vi "1D experiment kinect.vi"() -> ()   [LabVIEW 2011]
uses:
  <vilib>/Platform/TimedLoop/XDataNode/timing_clust.ctl
  <vilib>/Platform/TimedLoop/XDataNode/nitl_modes.ctl
  <vilib>/Platform/TimedLoop/XDataNode/wakeup.ctl
  <vilib>/Utility/inputDevices.llb/closeMouse.vi
  <vilib>/Utility/cursorutil.llb/Set Cursor (Cursor ID).vi
  <vilib>/Utility/inputDevices.llb/mouseAcquire.vi
  <vilib>/Utility/file.llb/Write To Spreadsheet File (DBL).vi
  <vilib>/Utility/file.llb/Write To Spreadsheet File (I64).vi
  <vilib>/Platform/TimedLoop/XDataNode/XDataNode.xnode
  <vilib>/Platform/TimedLoop/XDataNode/XDNodeRunTimeDep.lvlib
  User32.dll
  3D_Experiment/kinect-1-4/Kinect_API.lvlib
panel:
  in  "Far object filter 2":i32(slide)=26869 scale=0.0..4305.0
  out "click 2":bool
  in  "Replace with?":i32=60000
  out "stop":bool
  out "initial time":u32
  out "1D Experiment":cluster{"Y":dbl[], "Y":dbl[]}[](graph)
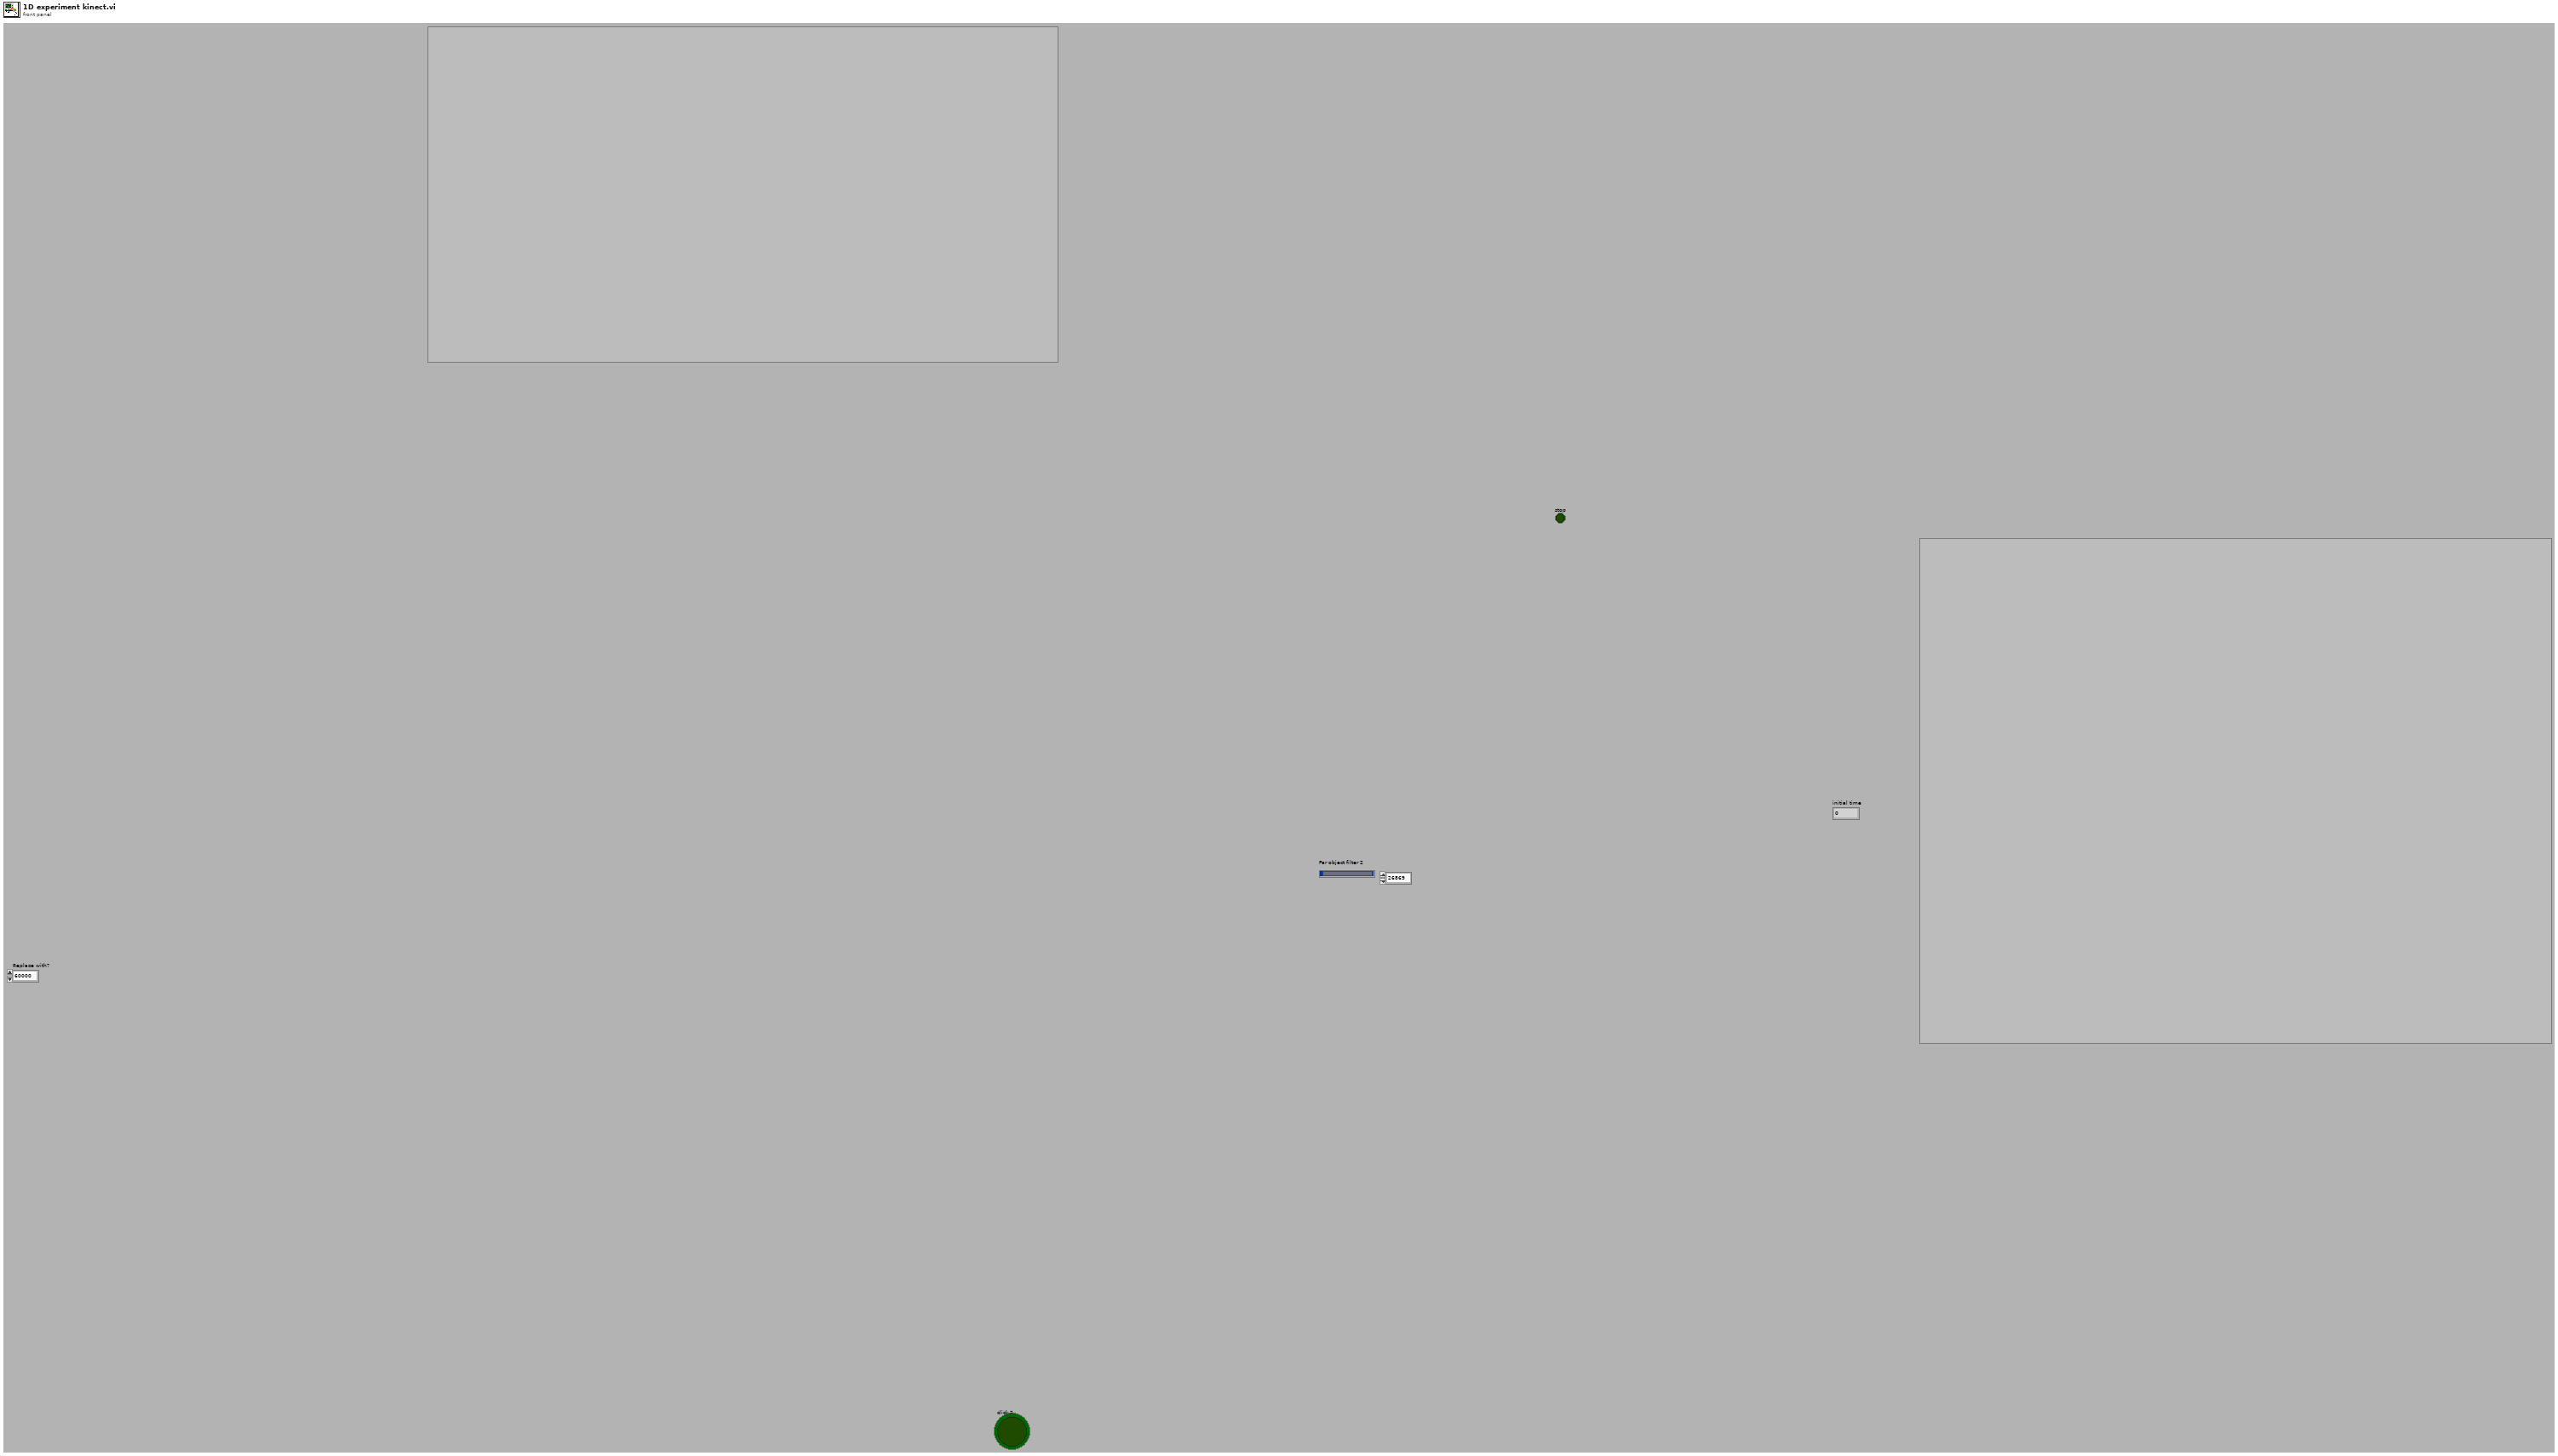
[diagram p1: front panel]
types:
  T1 = enum16{"open", "replace", "create", "open or create", "replace or create", "replace or create with confirmation"}
  T2 = typedef "XDNodeRunTimeDep.lvlib/timing_clust.ctl" = cluster{"Expected End [f-1]":u64, "Actual End [f-1]":u64, "Finished Late? [f-1]":bool, "Expected End [i-1]":u64, "Actual End [i-1]":u64, "Finished Late? [i-1]":bool, "Expected Start [i]":u64, "Actual Start [i]":u64, "Expected Start [f]":u64, "Actual Start [f]":u64, "Source Name":string, "Structure Name":string, "Period":i64, "Deadline":i64, "Offset":i64, "Start":i64, "Priority":i32, "Timeout":i32, "Mode":T3, "Wakeup Reason":T4, "Error":errorcluster, "Source Type":string, "Secondary Source Type":string, "Global End Time":u64, "Global Start Time":u64, "Frame Duration":u64, "Iteration Duration":u64, "Assigned CPU":i32, "I/O Scan Engine Mode":u32}
  T3 = typedef "XDNodeRunTimeDep.lvlib/nitl_modes.ctl" = enum32{"No Change", "Process missed periods, maintain original phase", "Discard missed periods, maintain original phase", "Process missed periods, ignore original phase", "Discard missed periods, ignore original phase"}
  T4 = typedef "XDNodeRunTimeDep.lvlib/wakeup.ctl" = enum32{"Normal", "Aborted", "Asynchronous wakeup", "Timing source error", "Timed loop error", "Timeout"}
  T5 = cluster{"Radius":dbl, "x0":dbl, "y0":dbl, "D":dbl, bool}
  T6 = typedef "LVAllMonitorsDisplayTypeDef.ctl" = cluster{"Bounds":cluster{"Left":i16, "Top":i16, "Right":i16, "Bottom":i16}, "Depth":i16}[]
  T7 = cluster{"Bounds":cluster{"Left":i16, "Top":i16, "Right":i16, "Bottom":i16}, "Depth":i16}
  T8 = cluster{"Left":i16, "Top":i16, "Right":i16, "Bottom":i16}
  T9 = cluster{"queue out":refnum<queue>, "queue out":refnum<queue>}
  T10 = cluster{"new reference":refnum<k24>, "DepthStream":refnum<k24>, "VideoStream":refnum<k24>, "Event Callback":refnum<k27>, "Event Callback":refnum<k27>}
  T11 = cluster{"Horizontal":i32, "Vertical":i32, "Scrolling":i32}
  T12 = cluster{"button 1":bool, "button 2":bool, "button 3":bool, "button 4":bool}
  T13 = typedef "LVPoint32TypeDef.ctl" = cluster{"Horizontal":i32, "Vertical":i32}
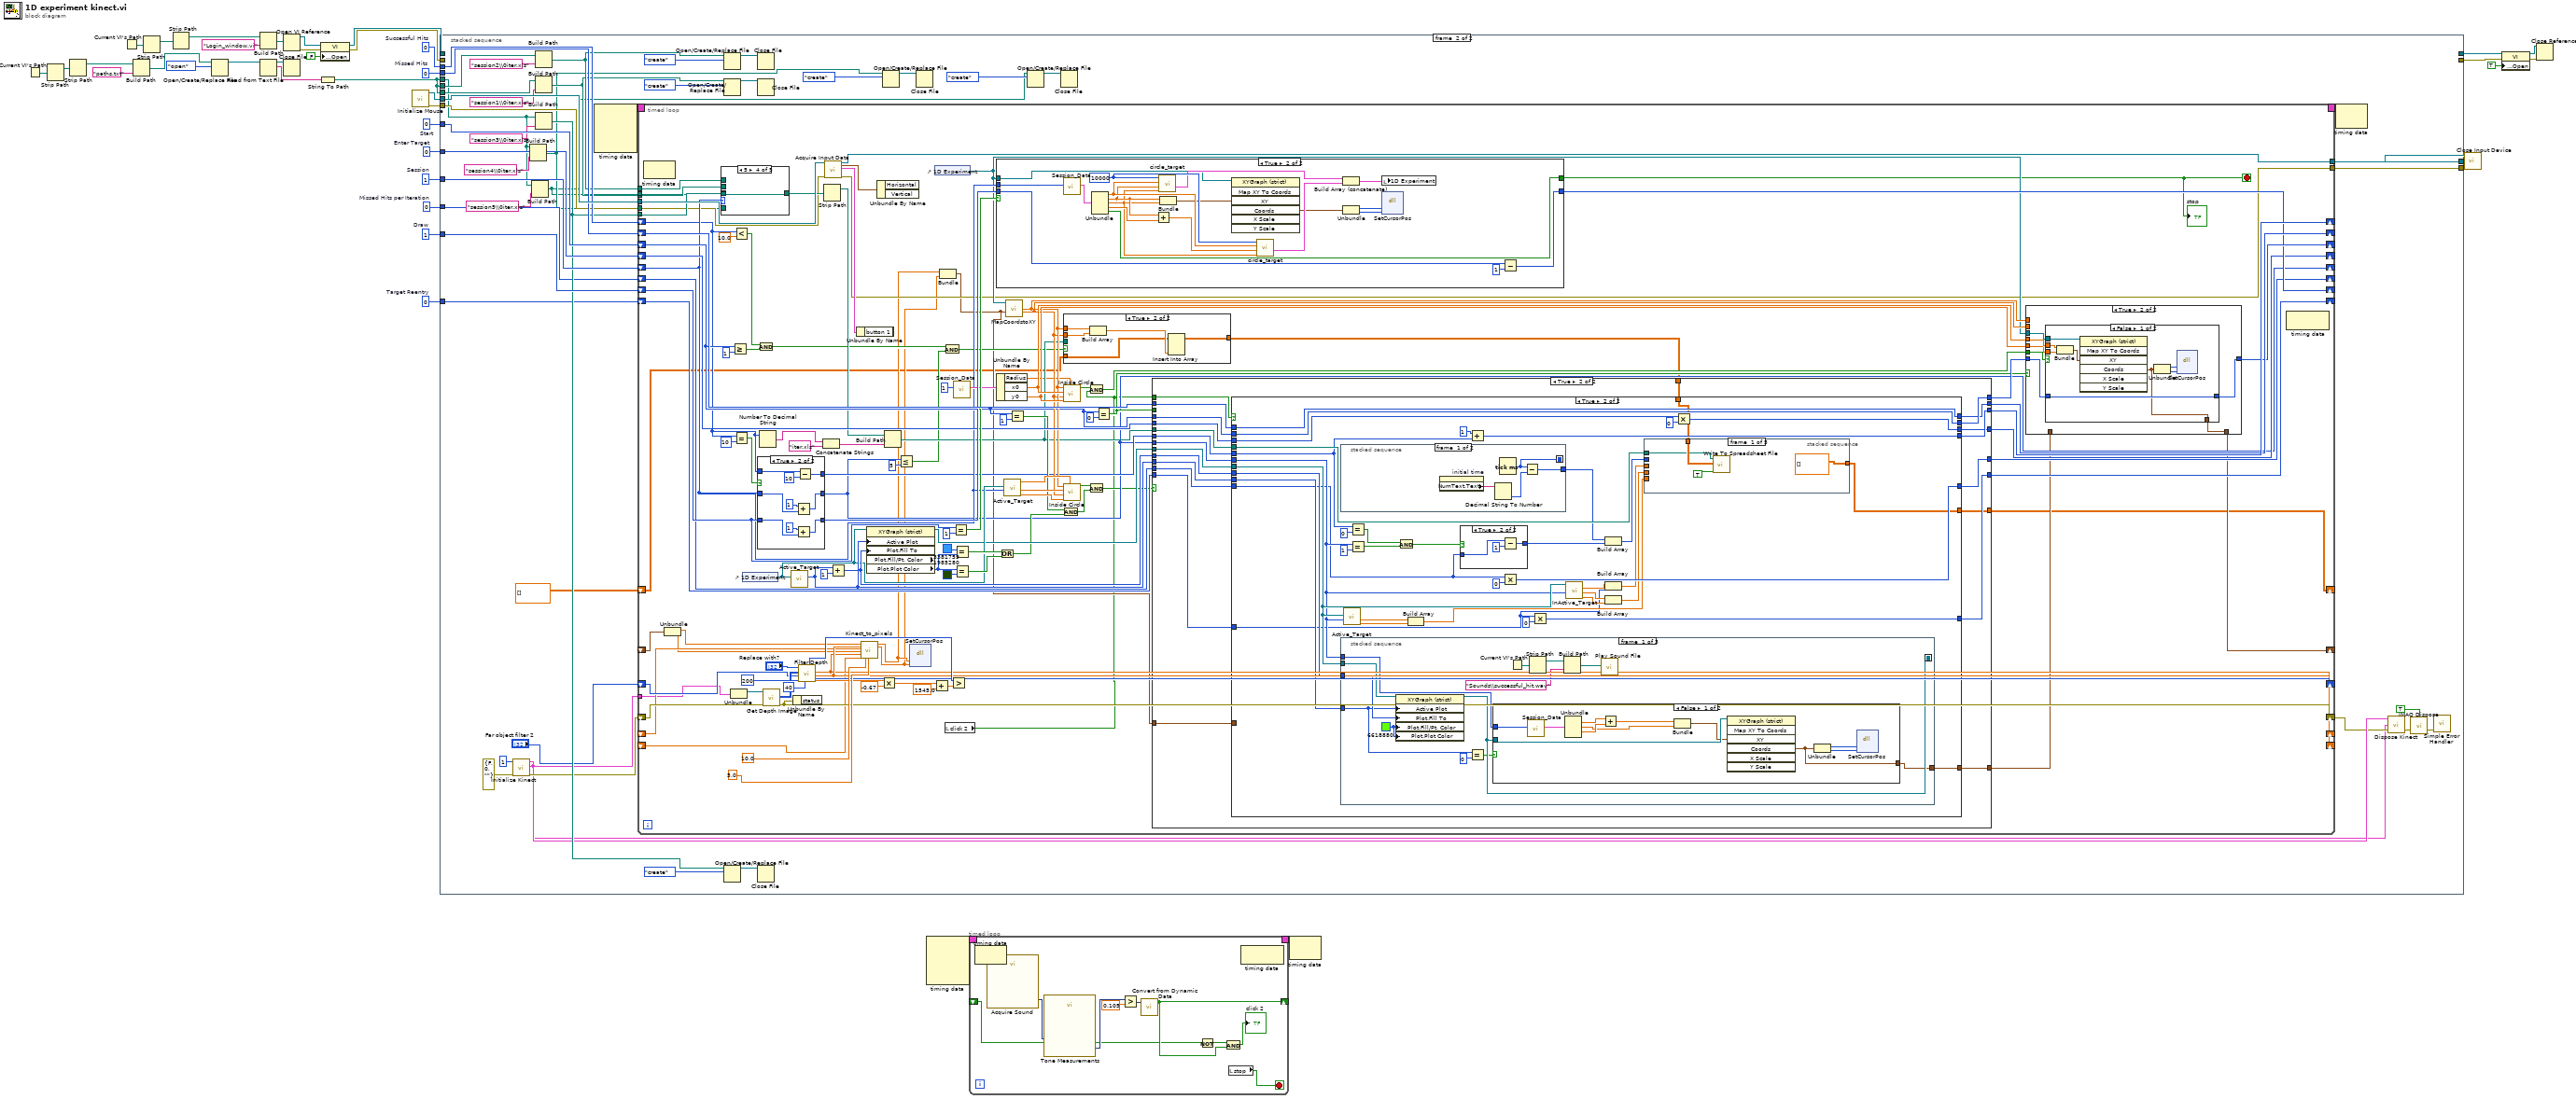
[diagram p0: block diagram]
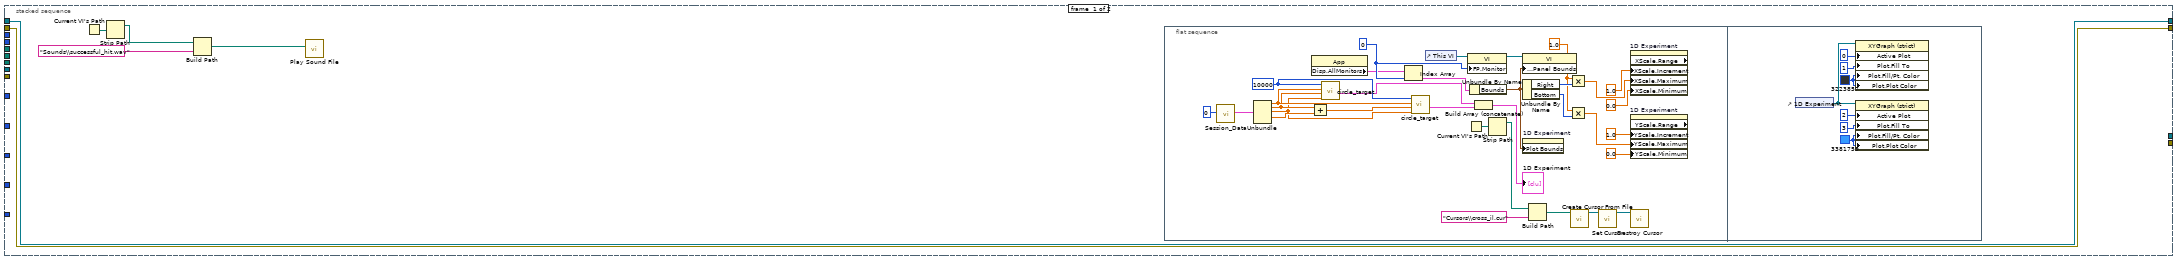
[diagram p2: hidden frame]
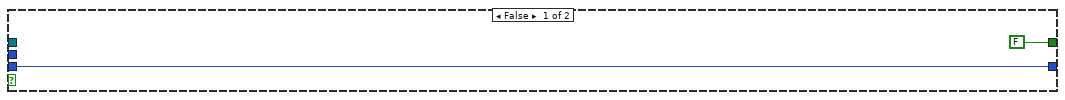
[diagram p8: hidden frame]
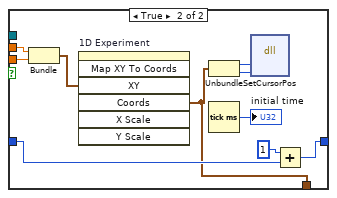
[diagram p10: hidden frame]
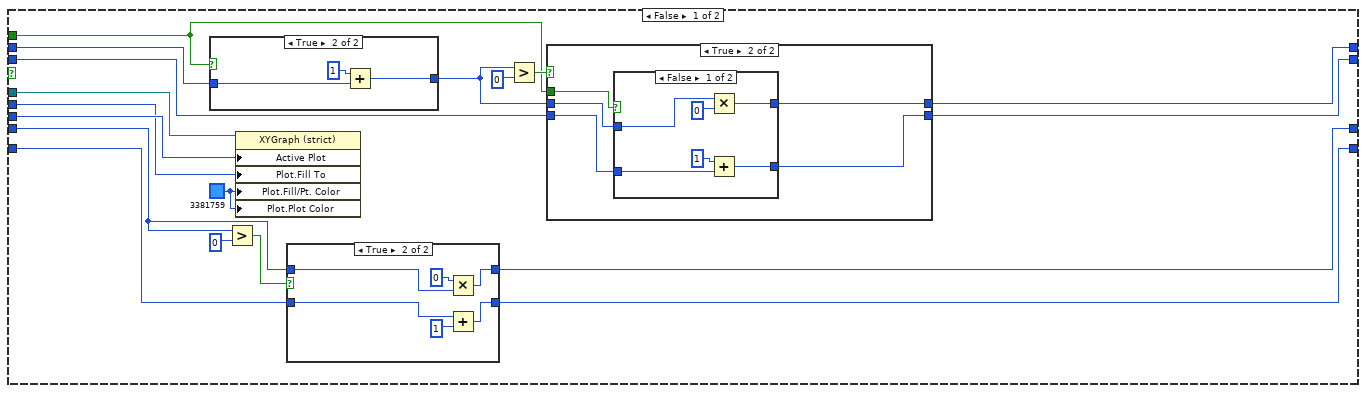
[diagram p13: hidden frame]
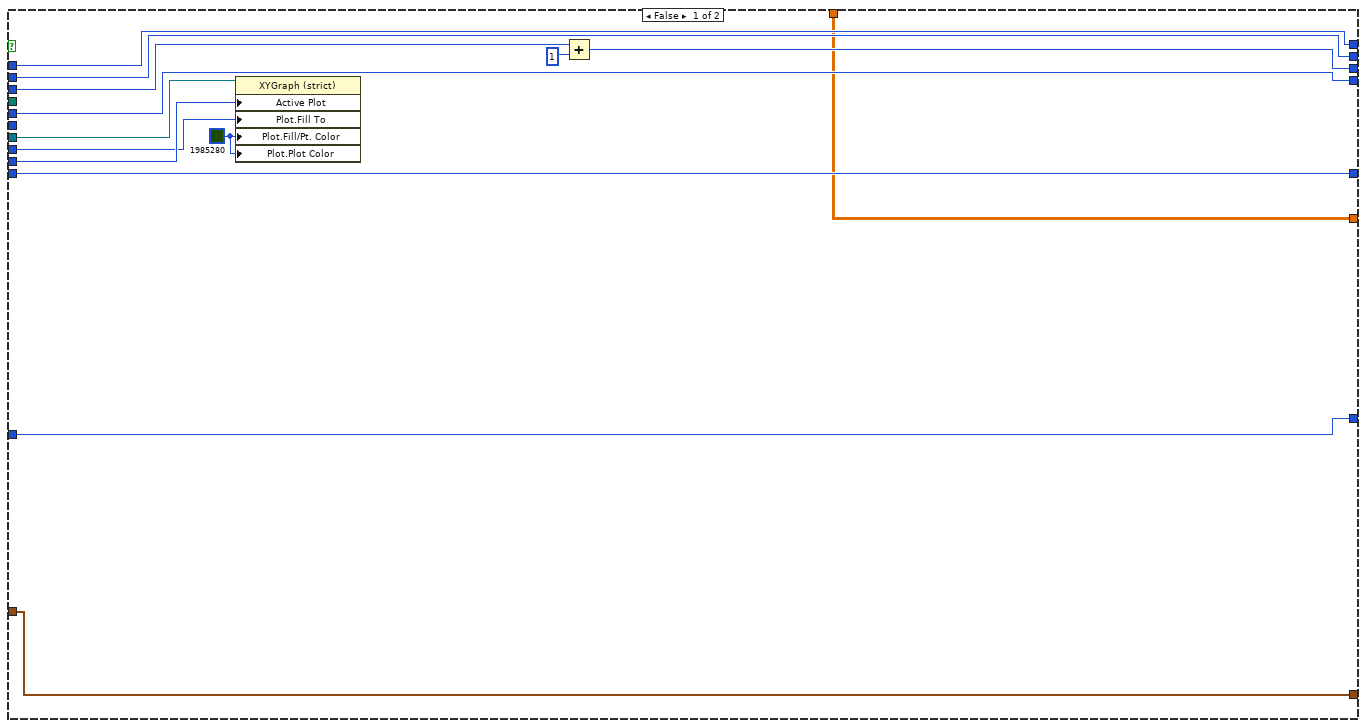
[diagram p18: hidden frame]
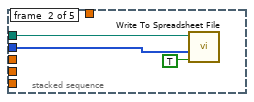
[diagram p20: hidden frame]
diagram:
  w5 = 0  # Target Reentry
  w6 = 0  # Missed Hits per Iteration
  w32 = 0  # Enter Target
  w33 = 1  # Draw
  w34 = 0  # Start
  w35 = 1  # Session
  w36 = 0  # Missed Hits
  w37 = 0  # Successful Hits
  n1 = Current VI's Path() -> (path=w14:path)
  n2 = Strip Path(path=w14) -> (stripped path=w9:path)  [unwired: 1 out]
  n3 = Strip Path(path=w9) -> (stripped path=w10:path)  [unwired: 1 out]
  n4 = Current VI's Path() -> (path=w17:path)
  n5 = Build Path(base path=w10, name or relative path="paths.txt") -> (appended path=w12:path)
  n6 = Strip Path(path=w17) -> (stripped path=w7:path)  [unwired: 1 out]
  n7 = Strip Path(path=w7) -> (stripped path=w8:path)  [unwired: 1 out]
  n8 = Open/Create/Replace File(file path (use dialog)=w12, operation (0:open)=T1."open") -> (refnum out=w30:refnum<file>)  [unwired: 4 in, 2 out]
  n9 = Build Path(base path=w8, name or relative path="Login_window.vi") -> (appended path=w15:path)
  n10 = Read from Text File(file (use dialog)=w30) -> (refnum out=w31:refnum<file>, text=w29:string)  [unwired: 3 in, 2 out]
  n11 = Open VI Reference(vi path=w15) -> (vi reference=w27:refnum<vi>, error out=w26:errorcluster)  [unwired: 5 in]
  n12 = Close File(refnum=w31) -> ()  [unwired: 1 in, 2 out]
  n13 = String To Path(string=w29) -> (path=w28:path)
  n14 = property class="VI"(reference=w27, error in=w26, "Front Panel Window:Open"=FALSE) -> (reference out=w24:refnum<vi>, error out=w23:errorcluster)
  n15 = call <vilib>:"Initialize Mouse.vi"() -> ("error out"=w4:errorcluster, "device ID"=w39:refnum<k1>)  [unwired: 1 in, 9 out]
  n16 = stacked-sequence {
    tunnel: w39 -> [_ w132]
    tunnel: [_ w131] -> w38
    tunnel: w37 -> [_ w130]
    tunnel: w36 -> [_ w129]
    tunnel: w35 -> [_ w125]
    tunnel: w34 -> [_ w128]
    tunnel: w33 -> [_ w127]
    tunnel: w32 -> [_ w126]
    tunnel: w28 -> [_ w115]
    tunnel: w28 -> [_ w122]
    tunnel: w28 -> [_ w102]
    tunnel: w24 -> [w41 _]
    tunnel: w23 -> [w40 _]
    tunnel: [w41 _] -> w19
    tunnel: [w40 _] -> w18
    tunnel: w6 -> [_ w108]
    tunnel: w5 -> [_ w107]
    tunnel: w4 -> [_ w106]
    tunnel: [_ w105] -> w3
    frame #0 {
      n17 = Current VI's Path() -> (path=w43:path)
      n18 = Strip Path(path=w43) -> (stripped path=w42:path)  [unwired: 1 out]
      n19 = Build Path(base path=w42, name or relative path="Sounds\\successful_hit.wav") -> (appended path=w44:path)
      n20 = call <vilib>:"Play Sound File.vi"("path"=w44) -> ()  [unwired: 9 in, 2 out]
      n21 = flat-sequence {
        frame #0 {
          w63 = 1.0 ("y")
          w68 = u16 0 ("Front Panel Window:Monitor")
          w77 = 10000
          n22 = call "Session_Data.vi"("Session"=0) -> ("output cluster"=w55:T5)  [unwired: 10 in]
          n23 = Unbundle(w55) -> ("Radius"=w75:dbl, "x0"=w53:dbl, "y0"=w52:dbl, "D"=w54:dbl)  [unwired: 1 out]
          n24 = Add(x=w53, y=w54) -> (x+y=w76:dbl)
          n25 = property class="App"() -> ("Disp.AllMonitors"=w67:T6)  [unwired: 2 in, 2 out]
          n26 = call "circle_target.vi"("y0"=w52, "x0"=w53, "Radius"=w75, "Pixels"=w77) -> ("Target plots"=w73:cluster{dbl[], dbl[]}[])  [unwired: 7 in]
          n27 = Index Array(array=w67, index=w68) -> (element=w69:T7)
          n28 = call "circle_target.vi"("y0"=w52, "x0"=w76, "Radius"=w75, "Pixels"=w77) -> ("Target plots"=w74:cluster{dbl[], dbl[]}[])  [unwired: 7 in]
          n29 = control-ref of="This VI"() -> (w70:refnum<vi>)
          n30 = Current VI's Path() -> (path=w51:path)
          n31 = property class="VI"(reference=w70, "FP.Monitor"=w68) -> (reference out=w66:refnum<vi>)  [unwired: 1 in, 1 out]
          n32 = Unbundle By Name(w69) -> ("Bounds"=w65:T8)
          n33 = Build Array (concatenate)(w73, w74) -> (→"1D Experiment":cluster{dbl[], dbl[]}[])
          n34 = Strip Path(path=w51) -> (stripped path=w50:path)  [unwired: 1 out]
          n35 = property class="VI"(reference=w66, "Front Panel Window:Panel Bounds"=w65) -> ()  [unwired: 1 in, 2 out]
          n36 = Unbundle By Name(w65) -> ("Right"=w64:i16, "Bottom"=w62:i16)
          n37 = property on="1D Experiment" class="XYGraph (strict)"("Plot Bounds"=w65) -> ()  [unwired: 2 in, 2 out]
          n38 = Build Path(base path=w50, name or relative path="Cursors\\cross_il.cur") -> (appended path=w48:path)
          n39 = Multiply(x=w63, y=w64) -> (x*y=w60:dbl)
          n40 = Multiply(x=w63, y=w62) -> (x*y=w57:dbl)
          n41 = call <vilib>:"Create Cursor From File.vi"("cursor file"=w48) -> ("cursor ID"=w47:refnum<k1>)  [unwired: 9 in, 1 out]
          n42 = call-poly <vilib>:"Set Cursor.vi"("cursor ID"=w47) -> ("previous cursor ID"=w46:refnum<k1>)  [unwired: 9 in, 1 out]
          n43 = property on="1D Experiment" class="XYGraph (strict)" props=["XScale", "Range", "XScale", "Increment", "XScale", "Maximum", "XScale", "Minimum"]("XScale.Increment"=1.0 ("X Scale.Range:Increment"), "XScale.Maximum"=w60, "XScale.Minimum"=0.0 ("X Scale.Range:Minimum")) -> ()  [unwired: 2 in, 3 out]
          n44 = property on="1D Experiment" class="XYGraph (strict)" props=["YScale", "Range", "YScale", "Increment", "YScale", "Maximum", "YScale", "Minimum"]("YScale.Increment"=1.0 ("Y Scale.Range:Increment"), "YScale.Maximum"=w57, "YScale.Minimum"=0.0 ("Y Scale.Range:Minimum")) -> ()  [unwired: 2 in, 3 out]
          n45 = call <vilib>:"Destroy Cursor.vi"("cursor ID"=w46) -> ()  [unwired: 9 in, 1 out]
        }
        frame #1 {
          w83 = u32 3381759
          w80 = u32 3223857
          n46 = control-ref of="1D Experiment"() -> (w84:refnum<vi>)
          n47 = property on="Property Node" class="XYGraph (strict)"(reference=w84, "Active Plot"=u32 0, "Plot.Fill To"=i16 1, "Plot.Fill/Pt. Color"=w80, "Plot.Plot Color"=w80) -> ()  [unwired: 1 in, 2 out]
          n48 = property on="Property Node" class="XYGraph (strict)"(reference=w84, "Active Plot"=u32 2, "Plot.Fill To"=i16 3, "Plot.Fill/Pt. Color"=w83, "Plot.Plot Color"=w83) -> ()  [unwired: 1 in, 2 out]
        }
      }
    }
    frame #1 {
      n49 = call "Initialize Kinect.vi"("error in (no error)"=errorcluster {"status"=FALSE, "code"=0, "source"=""}, "Buffer Size"=1) -> ("error out"=w93:errorcluster, "Queues Out"=w86:T9, "References"=w88:T10)  [unwired: 7 in]
      n50 = Build Path(base path=w102, name or relative path="session4\\0iter.xls") -> (appended path=w97:path)
      n51 = Build Path(base path=w102, name or relative path="session5\\0iter.xls") -> (appended path=w96:path)
      n52 = Build Path(base path=w122, name or relative path="session2\\0iter.xls") -> (appended path=w119:path)
      n53 = Build Path(base path=w115, name or relative path="session1\\0iter.xls") -> (appended path=w111:path)
      n54 = Build Path(base path=w102, name or relative path="session3\\0iter.xls") -> (appended path=w116:path)
      n55 = node-c288() -> (w110:T2)  [unwired: 4 in]
      n56 = timed-loop {
        tunnel: w132 -> [w236]
        tunnel: [w235] -> w131
        shift-right: [w233] -> _
        shift-left: w130 -> [w185]
        shift-right: [w231] -> _
        shift-left: w129 -> [w232]
        shift-right: [w176] -> _
        shift-left: w125 -> [w198]
        shift-right: [w223] -> _
        shift-left: w128 -> [w201]
        shift-right: [w217] -> _
        shift-left: w127 -> [w218]
        shift-right: [w213] -> _
        shift-left: w126 -> [w214]
        tunnel: w111 -> [w199]
        tunnel: w119 -> [w197]
        tunnel: w116 -> [w196]
        timing: w110 -> [_]
        timing-out: [_] -> w109
        shift-right: [w181] -> _
        shift-left: w108 -> [w183]
        shift-right: [w179] -> _
        shift-left: w107 -> [w180]
        tunnel: w106 -> [w171]
        tunnel: [w170] -> w105
        tunnel: w97 -> [w169]
        tunnel: w96 -> [w168]
        shift-right: [w153] -> _
        shift-left: "Far object filter 2" -> [w152]
        shift-right: [w151] -> w87
        shift-left: w93 -> [w150]
        shift-right: [w149] -> _
        shift-left: _ -> [w148]
        shift-right: [w147] -> _
        shift-left: _ -> [w146]
        tunnel: w86 -> [w145]
        shift-right: [w142] -> _
        shift-left: _ -> [w141]
        shift-right: [w133] -> _
        shift-left: dbl[][] [] -> [w135]
        stop <- w167 stop-if-true
        n57 = node-c288() -> ()  [unwired: 1 in, 1 out]
        n58 = Unbundle(w141) -> ("X_pixels"=w140:dbl, "Y_pixels"=w139:dbl)
        n59 = case shown="5" w198 {
          tunnel: w199 -> [_ _ _ _ w253]
          tunnel: [w249 w250 w251 w252 w253] -> w194
          tunnel: w197 -> [w249 _ _ _ _]
          tunnel: w196 -> [_ w250 _ _ _]
          tunnel: w169 -> [_ _ w251 _ _]
          tunnel: w168 -> [_ _ _ w252 _]
          frame 2 {
          }
          frame 3 {
          }
          frame 4 {
          }
          frame 5 {
          }
          frame 1, Default {
          }
        }
        n60 = Unbundle(w145) -> ("queue out"=w154:refnum<queue>)  [unwired: 1 out]
        n61 = Greater Or Equal?(x=w201, y=1) -> (x >= y?=w188:bool)
        n62 = Less?(x=w185, y=10.0) -> (x < y?=w187:bool)
        n63 = Equal?(x=w185, y=10) -> (x = y?=w229:bool)
        n64 = control-ref of="1D Experiment"() -> (w227:refnum<vi>)
        n65 = case shown="True" w229 {
          tunnel: w185 -> [w311 w320]
          tunnel: [w311 w318] -> w195
          tunnel: w198 -> [w310 w312]
          tunnel: [w310 w313] -> w176
          tunnel: w218 -> [w309 w316]
          tunnel: [w309 w314] -> w216
          frame False {
          }
          frame True {
            n66 = Add(x=1, y=w312) -> (x+y=w313:i32)
            n67 = Add(x=1, y=w316) -> (x+y=w314:i32)
            n68 = Subtract(x=w320, y=10) -> (x-y=w318:i32)
          }
        }
        n69 = And(x=w187, y=w188) -> (x .and. y?=w177:bool)
        n70 = Number To Decimal String(number=w185) -> (decimal integer string=w193:string)  [unwired: 1 in]
        n71 = call "Get Depth Image.vi"("error in (no error)"=w150, "queue in"=w154) -> ("error out"=w151:errorcluster, "Depth Image Pixels (U16)"=w156:u16[][])  [unwired: 6 in, 2 out]
        n72 = call "Active_Target.vi"("XYGraph Refnum"=w227) -> ("Active Plot"=w241:u32)  [unwired: 7 in, 3 out]
        n73 = Unbundle By Name(w151) -> ()  [unwired: 1 out]
        n74 = call "Filter Depth.vi"("Wall-Threshold"=40, "Y-Threshold"=200, "Far object filter"=w152, "Depth Image Pixels (U16)"=w156, "Replace with?"="Replace with?") -> ("average Z"=w162:dbl, "average Y"=w149:dbl, "average X"=w147:dbl, "New far object filter"=w153:i32, "Area"=w163:i32)  [unwired: 1 in, 1 out]
        n75 = Concatenate Strings(w193, "iter.xls" ("name or relative path")) -> (w191:string)
        n76 = Strip Path(path=w194) -> (stripped path=w190:path)  [unwired: 1 out]
        n77 = call-poly <vilib>:"Acquire Input Data.vi"("device ID"=w236, "error in (no error)"=w171) -> ("device ID"=w235:refnum<k1>, "axis info"=w234:T11, "button info"=w237:T12, "error out"=w170:errorcluster)  [unwired: 1 in, 13 out]
        n78 = Add(x=w241, y=u32 1) -> (x+y=w240:u32)
        n79 = Unbundle By Name(w237) -> ()  [unwired: 1 out]
        n80 = call "Kinect_to_pixels.vi"("previous_X_pixels"=w140, "current_X_kinect"=w149, "previous_X_kinect"=w148, "previous_Y_pixels"=w139, "current_Y_kinect"=w147, "previous_Y_kinect"=w146, "X_Y_speed"=10.0, "min_diff"=5.0) -> ("X_pixels"=w138:dbl, "Y_pixels"=w137:dbl)  [unwired: 8 in, 2 out]
        n81 = property on="Property Node" class="XYGraph (strict)" props=["Active Plot", "Plot", "Fill To", "Plot", "Fill/Pt. Color", "Plot", "Plot Color"](reference=w227, "Active Plot"=w241, "Plot.Fill To"=w240) -> (reference out=w220:refnum<vi>, "Plot.Plot Color"=w222:u32)  [unwired: 1 in, 2 out]
        n82 = Unbundle By Name(w234) -> ()  [unwired: 2 out]
        n83 = Multiply(x=w162, y=-0.67 ("x")) -> (x*y=w158:dbl)
        n84 = Build Path(base path=w190, name or relative path=w191) -> (appended path=w189:path)
        n85 = Less Or Equal?(x=w176, y=5) -> (x <= y?=w173:bool)
        n86 = dll-call lib="User32.dll" fn="SetCursorPos"(w138, w137) -> ()  [unwired: 6 in, 2 out]
        n87 = Add(x=w158, y=1545.0 ("x")) -> (x+y=w159:dbl)
        n88 = control-ref of="1D Experiment"() -> (w184:refnum<vi>)
        n89 = Bundle("X_pixels"=w138, "Y_pixels"=w137) -> (w143:cluster{"X_pixels":dbl, "Y_pixels":dbl})  [unwired: 1 in]
        n90 = And(x=w177, y=w173) -> (x .and. y?=w174:bool)
        n91 = local read "click 2"() -> (w136:bool)
        n92 = Greater?(x=w163, y=w159) -> ()  [unwired: 1 out]
        n93 = Equal?(x=w218, y=1) -> (x = y?=w215:bool)
        n94 = call "Session_Data.vi"("Session"=1) -> ("output cluster"=w207:T5)  [unwired: 10 in]
        n95 = Equal?(x=u32 3381759, y=w222) -> (x = y?=w244:bool)
        n96 = Equal?(x=w222, y=u32 1985280) -> (x = y?=w243:bool)
        n97 = case shown="True" w215 {
          tunnel: w198 -> [_ w270]
          tunnel: [w260 w280] -> w217
          tunnel: w216 -> [w260 w279]
          tunnel: [FALSE ("Valid") w269] -> w167
          tunnel: w184 -> [_ w265]
          frame False {
          }
          frame True {
            w278 = 10000
            n98 = call "Session_Data.vi"("Session"=w270) -> ("output cluster"=w273:T5)  [unwired: 10 in]
            n99 = Unbundle(w273) -> ("Radius"=w276:dbl, "x0"=w264:dbl, "y0"=w263:dbl, "D"=w272:dbl, w269:bool)
            n100 = Add(x=w264, y=w272) -> (x+y=w277:dbl)
            n101 = call "circle_target.vi"("y0"=w263, "x0"=w264, "Radius"=w276, "Pixels"=w278) -> ("Target plots"=w274:cluster{dbl[], dbl[]}[])  [unwired: 7 in]
            n102 = Bundle("x0"=w264, "y0"=w263) -> (w262:cluster{"x0":dbl, "y0":dbl})  [unwired: 1 in]
            n103 = invoke on="Invoke Node" class="XYGraph (strict)" method="Map XY To Coords"(reference=w265, "XY"=w262) -> ("Coords"=w268:T13)  [unwired: 5 in, 6 out]
            n104 = call "circle_target.vi"("y0"=w263, "x0"=w277, "Radius"=w276, "Pixels"=w278) -> ("Target plots"=w275:cluster{dbl[], dbl[]}[])  [unwired: 7 in]
            n105 = Build Array (concatenate)(w274, w275) -> (w271:cluster{dbl[], dbl[]}[])
            n106 = Unbundle(w268) -> ("Horizontal"=w267:i32, "Vertical"=w266:i32)
            n107 = local write "1D Experiment"(w271) -> ()
            n108 = dll-call lib="User32.dll" fn="SetCursorPos"(w267, w266) -> ()  [unwired: 6 in, 2 out]
            n109 = Subtract(x=w279, y=1) -> (x-y=w280:i32)
          }
        }
        "stop" <- w167
        n110 = Unbundle By Name(w207) -> ("Radius"=w178:dbl, "x0"=w206:dbl, "y0"=w205:dbl)
        n111 = Or(x=w244, y=w243) -> (x .or. y?=w211:bool)
        n112 = call "Active_Target.vi"("Session"=w198, "XYGraph Refnum"=w227) -> ("y0"=w238:dbl, "x0"=w239:dbl, "Radius"=w228:dbl)  [unwired: 6 in, 1 out]
        n113 = call "MapCoordstoXY.vi"("Coordinates"=w143, "XYGraph Refnum"=w184) -> ("Y(graph)"=w202:dbl, "X (graph)"=w203:dbl)  [unwired: 7 in]
        n114 = Equal?(x=w201, y=1) -> (x = y?=w209:bool)
        n115 = And(x=w209, y=w211) -> (x .and. y?=w208:bool)
        n116 = case shown="True" w174 {
          tunnel: w203 -> [_ w259]
          tunnel: w202 -> [_ w258]
          tunnel: w189 -> [_ _]
          tunnel: w135 -> [w254 w256]
          tunnel: [w254 w255] -> w134
          frame False {
          }
          frame True {
            n117 = Build Array(w259, w258) -> (w257:dbl[])
            n118 = Insert Into Array(array=w256, new element=w257) -> (w255:dbl[][])  [unwired: 2 in]
          }
        }
        n119 = call "Inside Circle.vi"("Radius"=w178, "y0"=w205, "y"=w202, "x0"=w206, "x"=w203) -> ("Inside Circle"=w225:bool)  [unwired: 6 in]
        n120 = call "Inside Circle.vi"("Radius"=w228, "y0"=w238, "y"=w202, "x0"=w239, "x"=w203) -> ("Inside Circle"=w210:bool)  [unwired: 6 in]
        n121 = And(x=w225, y=w136) -> (x .and. y?=w224:bool)
        n122 = And(x=w210, y=w208) -> (x .and. y?=w172:bool)
        n123 = Equal?(x=w201, y=0) -> (x = y?=w182:bool)
        n124 = case shown="True" w172 {
          tunnel: w136 -> [w331 w408]
          tunnel: w241 -> [w335 w405]
          tunnel: w240 -> [w334 w404]
          tunnel: w195 -> [w337 w407]
          tunnel: [w337 w406] -> w233
          tunnel: w232 -> [w336 w396]
          tunnel: [w328 w394] -> w231
          tunnel: w201 -> [w333 w403]
          tunnel: [w333 w402] -> w221
          tunnel: w220 -> [w332 w401]
          tunnel: w214 -> [w326 w400]
          tunnel: [w325 w399] -> w213
          tunnel: w176 -> [_ w398]
          tunnel: w189 -> [_ w397]
          tunnel: w183 -> [w330 w395]
          tunnel: w182 -> [w329 _]
          tunnel: [w327 w393] -> w181
          tunnel: w180 -> [w324 w392]
          tunnel: [w323 w391] -> w179
          tunnel: [w322 w390] -> w144
          tunnel: w143 -> [w322 w389]
          tunnel: w134 -> [w321 w388]
          tunnel: [w321 w387] -> w133
          frame False {
            n125 = case shown="True" w329 {
              tunnel: w336 -> [w354 w385]
              tunnel: w335 -> [w353 _]
              tunnel: w334 -> [w352 _]
              tunnel: w332 -> [w351 _]
              tunnel: w331 -> [w348 _]
              tunnel: w330 -> [w346 w386]
              tunnel: [w345 w385] -> w328
              tunnel: [w344 w386] -> w327
              tunnel: w326 -> [w341 w384]
              tunnel: [w340 w384] -> w325
              tunnel: w324 -> [w339 w383]
              tunnel: [w338 w383] -> w323
              frame False {
                w355 = u32 3381759
                n126 = case shown="True" w348 {
                  tunnel: w354 -> [w379 w382]
                  tunnel: [w379 w380] -> w347
                  frame False {
                  }
                  frame True {
                    n127 = Add(x=1, y=w382) -> (x+y=w380:i32)
                  }
                }
                n128 = Greater?(x=w341, y=0) -> (0:w342:bool)
                n129 = property on="Property Node" class="XYGraph (strict)"(reference=w351, "Active Plot"=w353, "Plot.Fill To"=w352, "Plot.Fill/Pt. Color"=w355, "Plot.Plot Color"=w355) -> ()  [unwired: 1 in, 2 out]
                n130 = case shown="True" w342 {
                  tunnel: w341 -> [w357 w363]
                  tunnel: [w357 w361] -> w340
                  tunnel: w339 -> [w356 w360]
                  tunnel: [w356 w358] -> w338
                  frame False {
                  }
                  frame True {
                    n131 = Multiply(x=0, y=w363) -> (x*y=w361:i32)
                    n132 = Add(x=w360, y=1) -> (x+y=w358:i32)
                  }
                }
                n133 = Greater?(x=w347, y=0) -> (0:w349:bool)
                n134 = case shown="True" w349 {
                  tunnel: [w364 w370] -> w344
                  tunnel: [w365 w369] -> w345
                  tunnel: w348 -> [_ w368]
                  tunnel: w347 -> [w365 w367]
                  tunnel: w346 -> [w364 w366]
                  frame False {
                  }
                  frame True {
                    n135 = case shown="False" w368 {
                      tunnel: [w375 w378] -> w370
                      tunnel: [w373 w377] -> w369
                      tunnel: w367 -> [w372 w377]
                      tunnel: w366 -> [w371 w378]
                      frame False {
                        n136 = Multiply(x=w372, y=0) -> (x*y=w373:i32)
                        n137 = Add(x=1, y=w371) -> (x+y=w375:i32)
                      }
                      frame True {
                      }
                    }
                  }
                }
              }
              frame True {
              }
            }
          }
          frame True {
            n138 = case shown="True" w408 {
              tunnel: w407 -> [w421 w436]
              tunnel: [w421 w456] -> w406
              tunnel: w405 -> [w420 w459]
              tunnel: w404 -> [w419 w458]
              tunnel: w403 -> [w417 w457]
              tunnel: [w417 w457] -> w402
              tunnel: w401 -> [w418 w443]
              tunnel: w400 -> [w413 w448]
              tunnel: [w414 w446] -> w399
              tunnel: w398 -> [_ w434]
              tunnel: w397 -> [_ w454]
              tunnel: w396 -> [w416 w452]
              tunnel: [w416 w452] -> w394
              tunnel: w395 -> [w415 w429]
              tunnel: [w415 w450] -> w393
              tunnel: w392 -> [w411 w427]
              tunnel: [w411 w445] -> w391
              tunnel: [w410 w425] -> w390
              tunnel: w389 -> [w410 _]
              tunnel: w388 -> [w409 w424]
              tunnel: [w409 w423] -> w387
              frame False {
                w422 = u32 1985280
                n139 = property on="Property Node" class="XYGraph (strict)"(reference=w418, "Active Plot"=w420, "Plot.Fill To"=w419, "Plot.Fill/Pt. Color"=w422, "Plot.Plot Color"=w422) -> ()  [unwired: 1 in, 2 out]
                n140 = Add(x=w413, y=1) -> (x+y=w414:i32)
              }
              frame True {
                n141 = stacked-sequence {
                  seq-local: [w481 _] -> [_ w485]
                  tunnel: [w482 _] -> w453
                  frame #0 {
                    n142 = property on="initial time" class="DigNum (strict)"() -> ("NumText.Text"=w484:string)  [unwired: 2 in, 2 out]
                    n143 = Decimal String To Number(string=w484) -> (number=w483:i32)  [unwired: 2 in, 1 out]
                    n144 = Tick Count (ms)() -> (millisecond timer value=w481:u32)
                    n145 = Subtract(x=w481, y=w483) -> (x-y=w482:u32)
                  }
                  frame #1 {
                    n146 = Number To Decimal String(number=w485) -> (decimal integer string=w486:string)  [unwired: 1 in]
                    n147 = property on="initial time" class="DigNum (strict)"("NumText.Text"=w486) -> ()  [unwired: 2 in, 2 out]
                  }
                }
                n148 = stacked-sequence {
                  seq-local: [w496 _ _] -> [_ w520 w529]
                  tunnel: w459 -> [w495 w521 w531]
                  tunnel: w458 -> [w498 _ w530]
                  tunnel: w443 -> [w497 _ _]
                  tunnel: w434 -> [w492 _ _]
                  tunnel: [w487 _ _] -> w425
                  frame #0 {
                    w499 = u32 6618880
                    n149 = property on="Property Node" class="XYGraph (strict)"(reference=w497, "Active Plot"=w495, "Plot.Fill To"=w498, "Plot.Fill/Pt. Color"=w499, "Plot.Plot Color"=w499) -> (reference out=w496:refnum<vi>)  [unwired: 1 in, 1 out]
                    n150 = Equal?(x=w495, y=u32 0) -> (x = y?=w493:bool)
                    n151 = case shown="False" w493 {
                      tunnel: w496 -> [w507 w513]
                      tunnel: w492 -> [w505 w517]
                      tunnel: [w500 w511] -> w487
                      frame False {
                        n152 = call "Session_Data.vi"("Session"=w505) -> ("output cluster"=w508:T5)  [unwired: 10 in]
                        n153 = Unbundle(w508) -> ("x0"=w503:dbl, "y0"=w501:dbl, "D"=w502:dbl)  [unwired: 2 out]
                        n154 = Add(x=w503, y=w502) -> (x+y=w504:dbl)
                        n155 = Bundle(w504, "y0"=w501) -> (w506:cluster{dbl, "y0":dbl})  [unwired: 1 in]
                        n156 = invoke on="Invoke Node" class="XYGraph (strict)" method="Map XY To Coords"(reference=w507, "XY"=w506) -> ("Coords"=w500:T13)  [unwired: 5 in, 6 out]
                        n157 = Unbundle(w500) -> ("Horizontal"=w510:i32, "Vertical"=w509:i32)
                        n158 = dll-call lib="User32.dll" fn="SetCursorPos"(w510, w509) -> ()  [unwired: 6 in, 2 out]
                      }
                      frame True {
                        n159 = call "Session_Data.vi"("Session"=w517) -> ("output cluster"=w516:T5)  [unwired: 10 in]
                        n160 = Unbundle(w516) -> ("x0"=w515:dbl, "y0"=w512:dbl)  [unwired: 3 out]
                        n161 = Bundle("x0"=w515, "y0"=w512) -> (w514:cluster{"x0":dbl, "y0":dbl})  [unwired: 1 in]
                        n162 = invoke on="Invoke Node" class="XYGraph (strict)" method="Map XY To Coords"(reference=w513, "XY"=w514) -> ("Coords"=w511:T13)  [unwired: 5 in, 6 out]
                        n163 = Unbundle(w511) -> ("Horizontal"=w519:i32, "Vertical"=w518:i32)
                        n164 = dll-call lib="User32.dll" fn="SetCursorPos"(w519, w518) -> ()  [unwired: 6 in, 2 out]
                      }
                    }
                    n165 = Current VI's Path() -> (path=w489:path)
                    n166 = Strip Path(path=w489) -> (stripped path=w488:path)  [unwired: 1 out]
                    n167 = Build Path(base path=w488, name or relative path="Sounds\\successful_hit.wav") -> (appended path=w490:path)
                    n168 = call <vilib>:"Play Sound File.vi"("path"=w490) -> ()  [unwired: 9 in, 2 out]
                  }
                  frame #1 {
                    w528 = u32 3381759
                    n169 = Subtract(x=w521, y=u32 2) -> (x-y=w525:u32)
                    n170 = To Long Integer(number=w525) -> (32bit integer=w524:i32)
                    n171 = Absolute Value(x=w524) -> (abs(x)=w522:i32)
                    n172 = Add(x=w522, y=u32 1) -> (x+y=w526:u32)
                    n173 = property on="Property Node" class="XYGraph (strict)"(reference=w520, "Active Plot"=w522, "Plot.Fill To"=w526, "Plot.Fill/Pt. Color"=w528, "Plot.Plot Color"=w528) -> ()  [unwired: 1 in, 2 out]
                  }
                  frame #2 {
                    w532 = u32 3223857
                    n174 = property on="Property Node" class="XYGraph (strict)"(reference=w529, "Active Plot"=w531, "Plot.Fill To"=w530, "Plot.Fill/Pt. Color"=w532, "Plot.Plot Color"=w532) -> ()  [unwired: 1 in, 2 out]
                  }
                }
                n175 = call "Active_Target.vi"("Session"=w434, "XYGraph Refnum"=w443) -> ("y0"=w438:dbl, "x0"=w439:dbl)  [unwired: 6 in, 2 out]
                n176 = Equal?(x=w436, y=0) -> (x = y?=w432:bool)
                n177 = Equal?(x=w434, y=1) -> (x = y?=w431:bool)
                n178 = And(x=w432, y=w431) -> (x .and. y?=w430:bool)
                n179 = Build Array(w439, w438) -> (w437:dbl[])
                n180 = case shown="True" w430 {
                  tunnel: w429 -> [w461 w464]
                  tunnel: [w461 w462] -> w428
                  frame False {
                  }
                  frame True {
                    n181 = Subtract(x=w464, y=1) -> (x-y=w462:i32)
                  }
                }
                n182 = Add(x=1, y=w436) -> (x+y=w456:i32)
                n183 = Multiply(x=w429, y=0) -> (x*y=w450:i32)
                n184 = Multiply(x=w427, y=0) -> (x*y=w445:i32)
                n185 = call "InActive_Target.vi"("Session"=w434, "XYGraph Refnum"=w443) -> ("y0"=w441:dbl, "x0"=w442:dbl, "Radius"=w426:dbl)  [unwired: 5 in, 1 out]
                n186 = Build Array(w453, w428) -> (w455:u32[])
                n187 = Build Array(w426, w427) -> (w444:dbl[])
                n188 = Build Array(w442, w441) -> (w440:dbl[])
                n189 = stacked-sequence {
                  tunnel: w455 -> [_ w471 _ _ _]
                  tunnel: w454 -> [w465 w469 w474 w477 w480]
                  tunnel: w444 -> [_ _ w473 _ _]
                  tunnel: w440 -> [_ _ _ w475 _]
                  tunnel: w437 -> [_ _ _ _ w478]
                  tunnel: [dbl[][] [] _ _ _ _] -> w423
                  tunnel: w424 -> [w466 _ _ _ _]
                  frame #0 {
                    n190 = call-poly <vilib>:"Write To Spreadsheet File.vi"("append to file? (new file:F)"=TRUE, "2D data"=w466, "file path (dialog if empty)"=w465) -> ()  [unwired: 5 in, 1 out]
                  }
                  frame #1 {
                    n191 = call-poly <vilib>:"Write To Spreadsheet File.vi"("append to file? (new file:F)"=TRUE, "1D data"=w471, "file path (dialog if empty)"=w469) -> ()  [unwired: 5 in, 1 out]
                  }
                  frame #2 {
                    n192 = call-poly <vilib>:"Write To Spreadsheet File.vi"("append to file? (new file:F)"=TRUE, "1D data"=w473, "file path (dialog if empty)"=w474) -> ()  [unwired: 5 in, 1 out]
                  }
                  frame #3 {
                    n193 = call-poly <vilib>:"Write To Spreadsheet File.vi"("append to file? (new file:F)"=TRUE, "1D data"=w475, "file path (dialog if empty)"=w477) -> ()  [unwired: 5 in, 1 out]
                  }
                  frame #4 {
                    n194 = call-poly <vilib>:"Write To Spreadsheet File.vi"("append to file? (new file:F)"=TRUE, "1D data"=w478, "file path (dialog if empty)"=w480) -> ()  [unwired: 5 in, 1 out]
                  }
                }
                n195 = Multiply(x=w448, y=0) -> (x*y=w446:i32)
              }
            }
          }
        }
        n196 = case shown="True" w182 {
          tunnel: w184 -> [_ w285]
          tunnel: w203 -> [_ _]
          tunnel: w202 -> [_ _]
          tunnel: w224 -> [_ w290]
          tunnel: w221 -> [w283 w289]
          tunnel: [w283 w288] -> w223
          tunnel: w206 -> [_ w287]
          tunnel: w205 -> [_ w286]
          tunnel: [w282 w284] -> w142
          tunnel: w144 -> [w282 _]
          frame False {
          }
          frame True {
            n197 = case shown="False" w290 {
              tunnel: w289 -> [w298 w308]
              tunnel: [w298 w306] -> w288
              tunnel: w287 -> [w297 w302]
              tunnel: w286 -> [w296 w301]
              tunnel: w285 -> [w292 _]
              tunnel: [w291 w299] -> w284
              frame False {
                n198 = Bundle("x0"=w297, "y0"=w296) -> (w295:cluster{"x0":dbl, "y0":dbl})  [unwired: 1 in]
                n199 = invoke on="Invoke Node" class="XYGraph (strict)" method="Map XY To Coords"(reference=w292, "XY"=w295) -> ("Coords"=w291:T13)  [unwired: 5 in, 6 out]
                n200 = Unbundle(w291) -> ("Horizontal"=w294:i32, "Vertical"=w293:i32)
                n201 = dll-call lib="User32.dll" fn="SetCursorPos"(w294, w293) -> ()  [unwired: 6 in, 2 out]
              }
              frame True {
                n202 = Bundle("x0"=w302, "y0"=w301) -> (w305:cluster{"x0":dbl, "y0":dbl})  [unwired: 1 in]
                n203 = invoke on="1D Experiment" class="XYGraph (strict)" method="Map XY To Coords"("XY"=w305) -> ("Coords"=w299:T13)  [unwired: 6 in, 6 out]
                n204 = Unbundle(w299) -> ("Horizontal"=w304:i32, "Vertical"=w303:i32)
                n205 = Tick Count (ms)() -> (millisecond timer value=→"initial time":u32)
                n206 = dll-call lib="User32.dll" fn="SetCursorPos"(w304, w303) -> ()  [unwired: 6 in, 2 out]
                n207 = Add(x=1, y=w308) -> (x+y=w306:i32)
              }
            }
          }
        }
        n208 = node-c288() -> ()  [unwired: 1 in, 1 out]
      }
      n209 = Open/Create/Replace File(file path (use dialog)=w119, operation (0:open)=T1."create") -> (refnum out=w121:refnum<file>)  [unwired: 4 in, 2 out]
      n210 = Open/Create/Replace File(file path (use dialog)=w111, operation (0:open)=T1."create") -> (refnum out=w113:refnum<file>)  [unwired: 4 in, 2 out]
      n211 = Open/Create/Replace File(file path (use dialog)=w116, operation (0:open)=T1."create") -> (refnum out=w118:refnum<file>)  [unwired: 4 in, 2 out]
      n212 = Close File(refnum=w121) -> ()  [unwired: 1 in, 2 out]
      n213 = Close File(refnum=w113) -> ()  [unwired: 1 in, 2 out]
      n214 = Close File(refnum=w118) -> ()  [unwired: 1 in, 2 out]
      n215 = Open/Create/Replace File(file path (use dialog)=w97, operation (0:open)=T1."create") -> (refnum out=w101:refnum<file>)  [unwired: 4 in, 2 out]
      n216 = Close File(refnum=w101) -> ()  [unwired: 1 in, 2 out]
      n217 = Open/Create/Replace File(file path (use dialog)=w96, operation (0:open)=T1."create") -> (refnum out=w99:refnum<file>)  [unwired: 4 in, 2 out]
      n218 = Close File(refnum=w99) -> ()  [unwired: 1 in, 2 out]
      n219 = node-c288(w109) -> ()  [unwired: 1 out]
      n220 = call "Dispose Kinect.vi"("error in (no error)"=w87, "Queues In"=w86, "References"=w88) -> ("error out"=w89:errorcluster)  [unwired: 2 in]
      n221 = call "IMAQ Dispose"("All Images? (No)"=TRUE, "error in (no error)"=w89) -> ("error out"=w90:errorcluster)  [unwired: 4 in]
      n222 = call <vilib>:"Simple Error Handler.vi"("error in (no error)"=w90) -> ()  [unwired: 4 in, 5 out]
    }
  }
  n223 = node-c288() -> (w2:T2)  [unwired: 4 in]
  n224 = timed-loop {
    shift-right: [w537] -> _
    shift-left: _ -> [w536]
    timing: w2 -> [_]
    timing-out: [_] -> w1
    stop <- w535 stop-if-true
    n225 = node-c288() -> ()  [unwired: 1 in, 1 out]
    n226 = call "Acquire Sound"() -> ("Data"=w543:dynamicdata)  [unwired: 18 in, 1 out]
    n227 = call "Tone Measurements"("Signals"=w543) -> ("Amplitude"=w542:dynamicdata)  [unwired: 9 in, 1 out]
    n228 = Greater?(x=w542, y=0.105) -> (0:w540:dynamicdata)
    n229 = call "Convert from Dynamic Data"("Dynamic Data Type"=w540) -> ("Scalar"=w537:bool)  [unwired: 3 in]
    n230 = Not(x=w536) -> (.not. x?=w539:bool)
    n231 = And(x=w539, y=w537) -> (x .and. y?=→"click 2":bool)
    n232 = local read "stop"() -> (w535:bool)
    n233 = node-c288() -> ()  [unwired: 1 in, 1 out]
  }
  n234 = node-c288(w1) -> ()  [unwired: 1 out]
  n235 = call-poly <vilib>:"Close Input Device.vi"("error in (no error)"=w3, "device ID"=w38) -> ()  [unwired: 9 out]
  n236 = property class="VI"(reference=w19, error in=w18, "Front Panel Window:Open"=TRUE) -> (reference out=w21:refnum<vi>, error out=w20:errorcluster)
  n237 = Close Reference(reference=w21, error in (no error)=w20) -> ()  [unwired: 1 out]
